vi "synch.vi"() -> ()   [LabVIEW 2014]
uses:
  <vilib>/Analysis/_algsub.llb/Real Vector Norm.vi
  <vilib>/Analysis/NI_AALPro.lvlib
panel:
  in  "Numeric":i32=500
  out "Waveform Graph":dbl[](graph)
  in  "X 2":dbl[](array[numeric])=[0.1, 0.1, 0.1]
  in  "X":dbl[](array[numeric])=[0.1, 0.1, 0.1]
  in  "A":dbl[](array[numeric])=[10.0, 28.0, 2.666666]
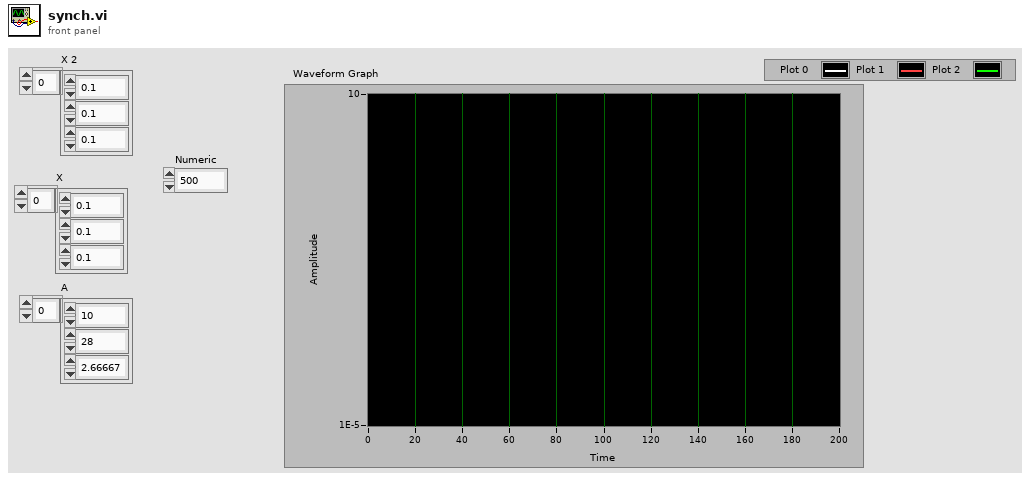
[diagram p1: front panel]
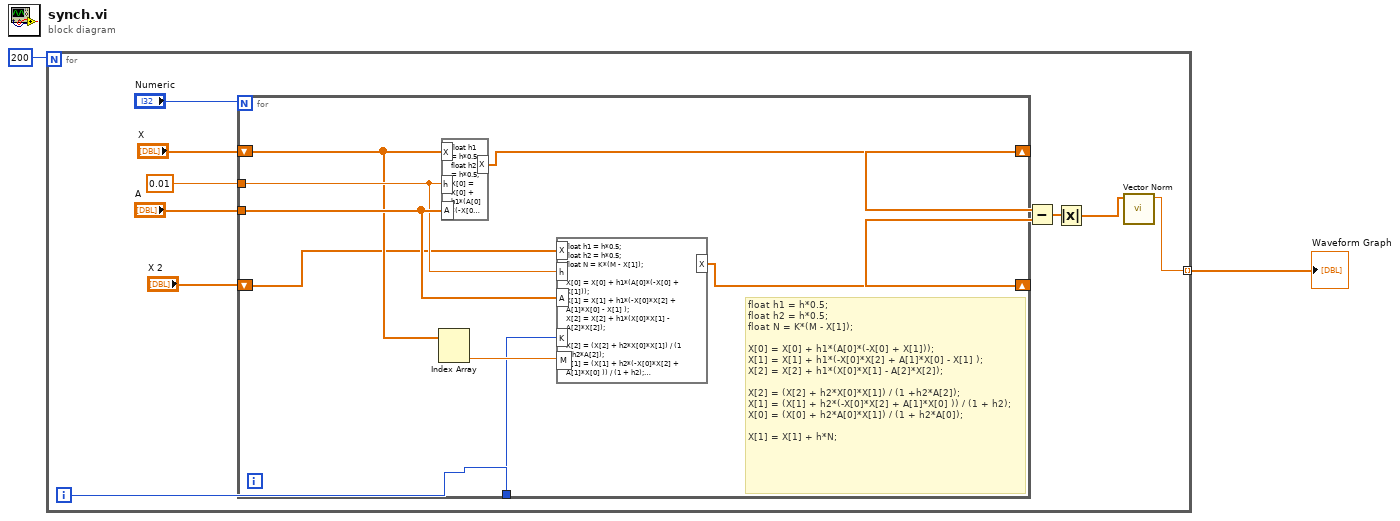
[diagram p0: block diagram]
diagram:
  n1 = for {
    N: 200 -> [_]
    tunnel: [w5] -> w1 mode=indexing
    i -> [w4]
    n2 = for {
      N: "Numeric" -> [_]
      tunnel: "A" -> [w21]
      shift-right: [w15] -> w8
      shift-left: "X" -> [w19]
      tunnel: 0.01 -> [w20]
      shift-right: [w14] -> w7
      shift-left: "X 2" -> [w17]
      tunnel: w4 -> [w16]
      # "float h1 = h*0.5;\nfloat h2 = h*0.5;\nfloat N = K*(M - X[1]);\n\nX[0] = X[0] + h1*(A[0]*(-X[0] + X[1]));\nX[1] = X[1] + h1*(-X[0]*X[2] + A[1]*X[0] - X[1] );\nX[2] = X[2] + h1*(X[0]*X[1] - A[2]*X[2]);\n\nX[2] = (X[2] + h2*X[0]*X[1]) / (1 +h2*A[2]);\nX[1] = (X[1] + h2*(-X[0]*X[2] + A[1]*X[0] )) / (1 + h2);\nX[0] = (X[0] + h2*A[0]*X[1]) / (1 + h2*A[0]);\n\nX[1] = X[1] + h*N;"
      n3 = Index Array(array=w19) -> (element #2=w18:dbl)  [unwired: 2 in, 1 out]
      n4 = formula code="float h1 = h*0.5;\nfloat h2 = h*0.5;\nX[0] = X[0] + h1*(A[0]*(-X[0] + X[1]));\nX[1] = X[1] + h1*(-X[0]*X[2] + A[1]*X[0] - X[1]);\nX[2] = X[2] + h1*(X[0]*X[1] - A[2]*X[2]);\n\nX[2] = (X[2] + h2*X[0]*X[1]) / (1 +h2*A[2]);\nX[1] = (X[1] + h2*(-X[0]*X[2] + A[1]*X[0])) / (1 + h2);\nX[0] = (X[0] + h2*A[0]*X[1]) / (1 + h2*A[0]);"("h"=w20, "X"=w19, "A"=w21) -> ("X"=w15:dbl[])
      n5 = formula code="float h1 = h*0.5;\nfloat h2 = h*0.5;\nfloat N = K*(M - X[1]);\n\nX[0] = X[0] + h1*(A[0]*(-X[0] + X[1]));\nX[1] = X[1] + h1*(-X[0]*X[2] + A[1]*X[0] - X[1] );\nX[2] = X[2] + h1*(X[0]*X[1] - A[2]*X[2]);\n\nX[2] = (X[2] + h2*X[0]*X[1]) / (1 +h2*A[2]);\nX[1] = (X[1] + h2*(-X[0]*X[2] + A[1]*X[0] )) / (1 + h2);\nX[0] = (X[0] + h2*A[0]*X[1]) / (1 + h2*A[0]);\n\nX[1] = X[1] + h*N;" ("Formula Node 2")("h"=w20, "X"=w17, "A"=w21, "K"=w16, "M"=w18) -> ("X"=w14:dbl[])
    }
    n6 = Subtract(x=w8, y=w7) -> (x-y=w9:dbl[])
    n7 = Absolute Value(x=w9) -> (abs(x)=w6:dbl[])
    n8 = call-poly <vilib>:"Vector Norm.vi"("Input Vector"=w6) -> ("norm"=w5:dbl)  [unwired: 9 in, 1 out]
  }
  "Waveform Graph" <- w1
